vi "pulses2commands_rabi.vi"(10 "MW_width":dbl, 11 "Rabi_parameters":T1) -> (3 "Array out":T2(array[cluster]))   [LabVIEW 2018]
panel:
  in  "Repetitions":i32
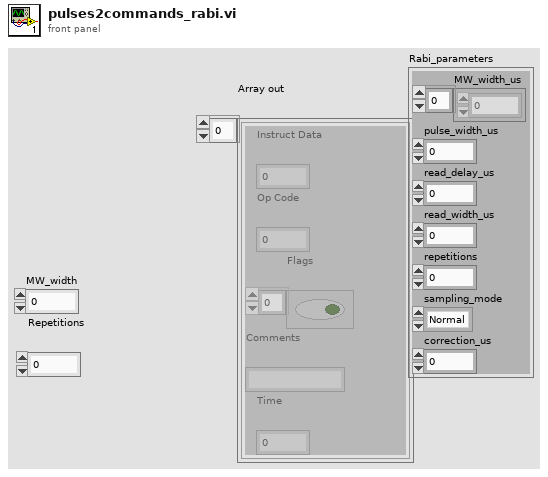
[diagram p1: front panel]
types:
  T1 = cluster{"MW_width_us":dbl[], "pulse_width_us":dbl, "read_delay_us":dbl, "read_width_us":dbl, "repetitions":i32, "sampling_mode":enum16{"Normal", "Sweep"}, "correction_us":dbl}
  T2 = cluster{"Instruct Data":i32, "Op Code":i32, "Flags":bool[], "Comments":string, "Time":dbl}[]
  T3 = cluster{"Instruct Data":i32, "Op Code":i32, "Flags":bool[], "Comments":string, "Time":dbl}
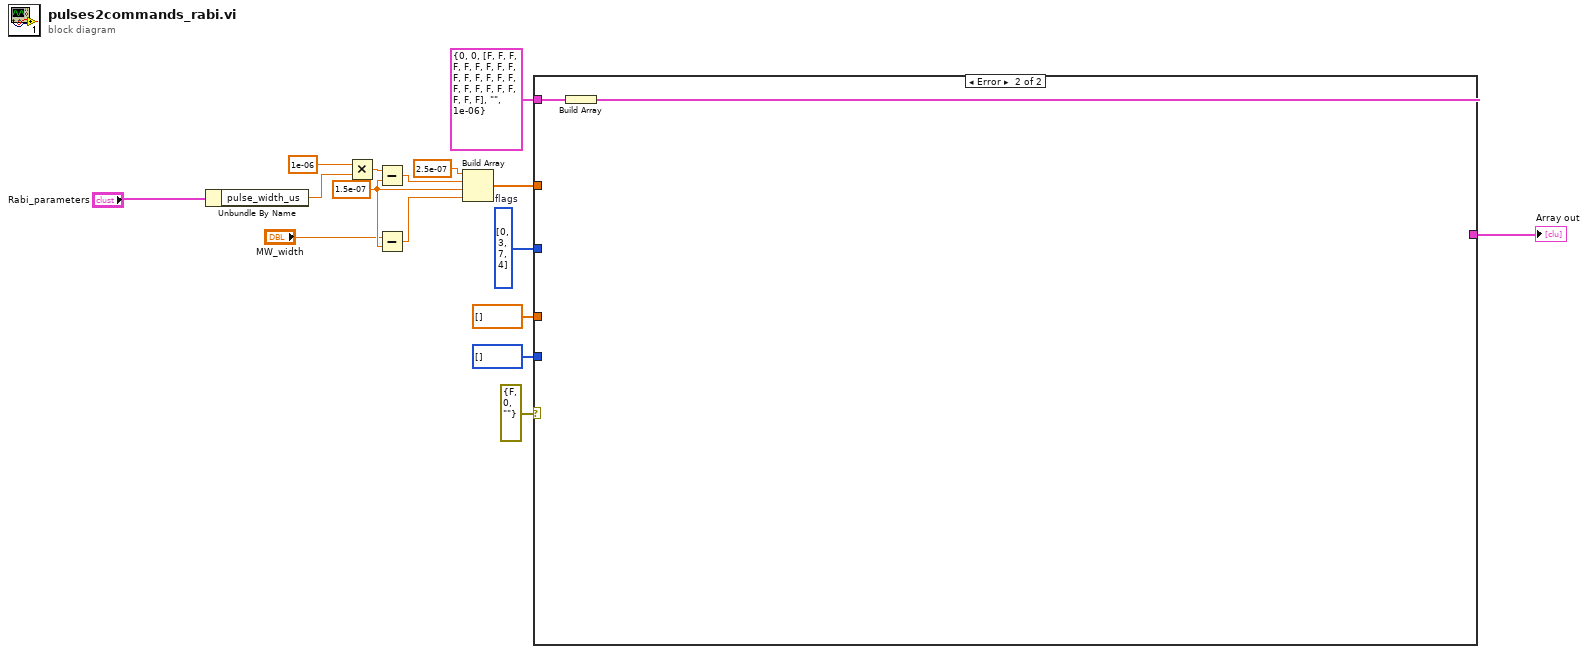
[diagram p0: block diagram]
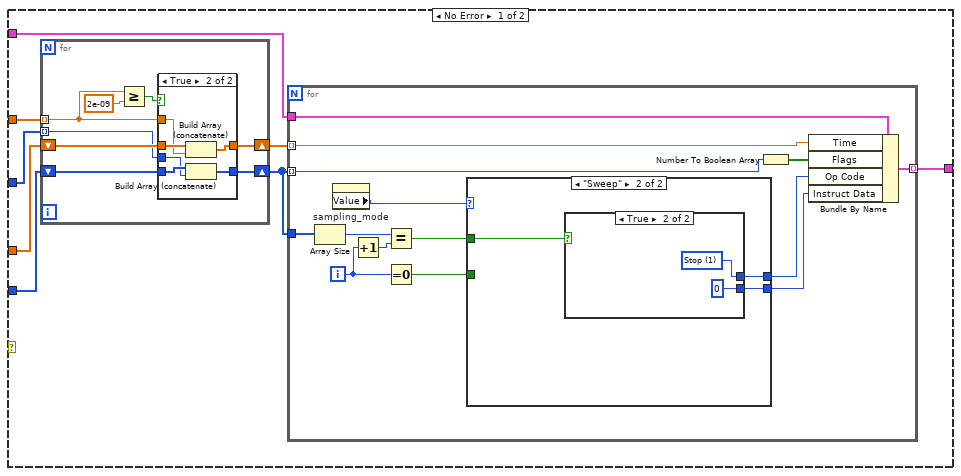
[diagram p2: hidden frame]
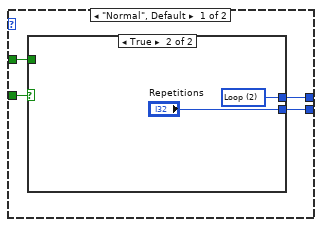
[diagram p3: hidden frame]
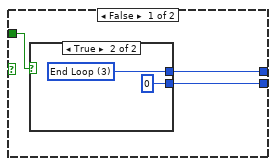
[diagram p4: hidden frame]
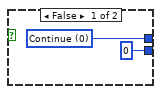
[diagram p5: hidden frame]
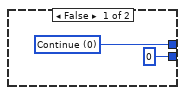
[diagram p6: hidden frame]
diagram:
  w7 = 1.5e-07
  w15 = u8[] [0, 3, 7, 4]  # flags
  n1 = Unbundle By Name("Rabi_parameters") -> ("pulse_width_us"=w2:dbl)
  n2 = Multiply(x=1e-06, y=w2) -> (x*y=w1:dbl)
  n3 = Subtract(x=w1, y=w7) -> (x-y=w8:dbl)
  n4 = Subtract(x="MW_width", y=w7) -> (x-y=w6:dbl)
  n5 = Build Array(2.5e-07, w8, w7, w6) -> (w11:dbl[])
  n6 = case shown="Error" errorcluster {"status"=FALSE, "code"=0, "source"=""} ("error constant") {
    tunnel: w11 -> [w24 _]
    tunnel: dbl[] [] -> [w23 _]
    tunnel: u8[] [] -> [w22 _]
    tunnel: w15 -> [w21 _]
    tunnel: T3 {"Instruct Data"=0, "Op Code"=0, "Flags"=[FALSE, FALSE, FALSE, FALSE, FALSE, FALSE, FALSE, FALSE, FALSE, FALSE, FALSE, FALSE, FALSE, FALSE, FALSE, FALSE, FALSE, FALSE, FALSE, FALSE, FALSE, FALSE, FALSE, FALSE], "Comments"="", "Time"=1e-06} ("PB Instruction") -> [w20 w75]
    tunnel: [w17 w76] -> w10
    frame No Error {
      n7 = for {
        tunnel: w24 -> [w63] mode=indexing
        shift-right: [w59] -> w18
        shift-left: w22 -> [w62]
        shift-right: [w60] -> w19
        shift-left: w23 -> [w64]
        tunnel: w21 -> [w61] mode=indexing
        n8 = Greater Or Equal?(x=w63, y=2e-09) -> (x >= y?=w66:bool)
        n9 = case shown="True" w66 {
          tunnel: w64 -> [w68 w74]
          tunnel: w63 -> [_ w73]
          tunnel: w62 -> [w67 w72]
          tunnel: w61 -> [_ w71]
          tunnel: [w68 w70] -> w60
          tunnel: [w67 w69] -> w59
          frame False {
          }
          frame True {
            n10 = Build Array (concatenate)(w74, w73) -> (w70:dbl[])
            n11 = Build Array (concatenate)(w72, w71) -> (w69:u8[])
          }
        }
      }
      n12 = for {
        tunnel: w20 -> [w37]
        tunnel: w19 -> [w29] mode=indexing
        tunnel: w18 -> [w31]
        tunnel: w18 -> [w28] mode=indexing
        tunnel: [w26] -> w17 mode=indexing
        i -> [w32]
        n13 = Array Size(array=w31) -> (size(s)=w30:i32)
        n14 = property on="sampling_mode" class="Enum (strict)"() -> ("Value"=w25:enum16{"Normal", "Sweep"})  [unwired: 2 in, 2 out]
        n15 = Increment(x=w32) -> (x+1=w33:i32)
        n16 = Equal?(x=w30, y=w33) -> (x = y?=w34:bool)
        n17 = Equal To 0?(x=w32) -> (x = 0?=w38:bool)
        n18 = case shown="\"Sweep\"" w25 {
          tunnel: w38 -> [w42 _]
          tunnel: [w41 w52] -> w36
          tunnel: [w40 w53] -> w35
          tunnel: w34 -> [w39 w54]
          frame "Normal", Default {
            n19 = case shown="True" w42 {
              tunnel: [w44 "Repetitions"] -> w41
              tunnel: [w43 w51] -> w40
              tunnel: w39 -> [w45 _]
              frame False {
                n20 = case shown="True" w45 {
                  tunnel: [0 0] -> w44
                  tunnel: [w47 w48] -> w43
                  frame False {
                    w47 = 0 items=["Continue", "Stop", "Loop", "End Loop", "JSR", "RTS", "Branch", "Long Delay", "Wait"] ("Op Code")
                  }
                  frame True {
                    w48 = 3 items=["Continue", "Stop", "Loop", "End Loop", "JSR", "RTS", "Branch", "Long Delay", "Wait"] ("Op Code 2")
                  }
                }
              }
              frame True {
                w51 = 2 items=["Continue", "Stop", "Loop", "End Loop", "JSR", "RTS", "Branch", "Long Delay", "Wait"] ("Op Code 2")
              }
            }
          }
          frame "Sweep" {
            n21 = case shown="True" w54 {
              tunnel: [w56 w58] -> w53
              tunnel: [0 0] -> w52
              frame False {
                w56 = 0 items=["Continue", "Stop", "Loop", "End Loop", "JSR", "RTS", "Branch", "Long Delay", "Wait"] ("Op Code 2")
              }
              frame True {
                w58 = 1 items=["Continue", "Stop", "Loop", "End Loop", "JSR", "RTS", "Branch", "Long Delay", "Wait"] ("Op Code 2")
              }
            }
          }
        }
        n22 = Number To Boolean Array(number=w28) -> (Boolean array=w27:bool[])
        n23 = Bundle By Name(cluster=w37, "Time"=w29, "Flags"=w27, "Op Code"=w35, "Instruct Data"=w36) -> (w26:T3)
      }
    }
    frame Error {
      n24 = Build Array(w75) -> (w76:T2)
    }
  }
  "Array out" <- w10
